vi "acquisitionSplitVolumes.vi"(4 "i-th volume":i32 min=0, 5 "volumeFirstFrame (from DAQ)":u32[](array[numeric]), 6 "frameCount (from Hamamatsu)":i32[](array[numeric]), 7 "frames":u16[][][](array[numeric])) -> (0 "numberOfFrames":i32, 1 "indexFirstFrame":i32, 2 "croppedFrameCount":u32[](array[numeric]), 3 "croppedFrames (volume)":u16[][][](array[numeric]))   [LabVIEW 2017]
doc: "Crop a single volume out of a continuous recording of frames, based on the two frame counts\nand the differentiator of the piezo monitor."
uses:
  globalUtilities.vi
panel:
  # "Crop a single volume out of a continuous recording of frames, based on the two frame counts\nand the differentiator of the piezo monitor."
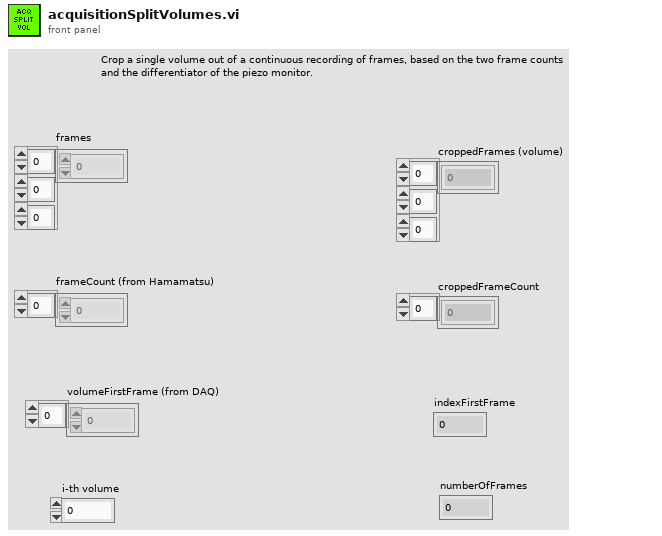
[diagram p1: front panel]
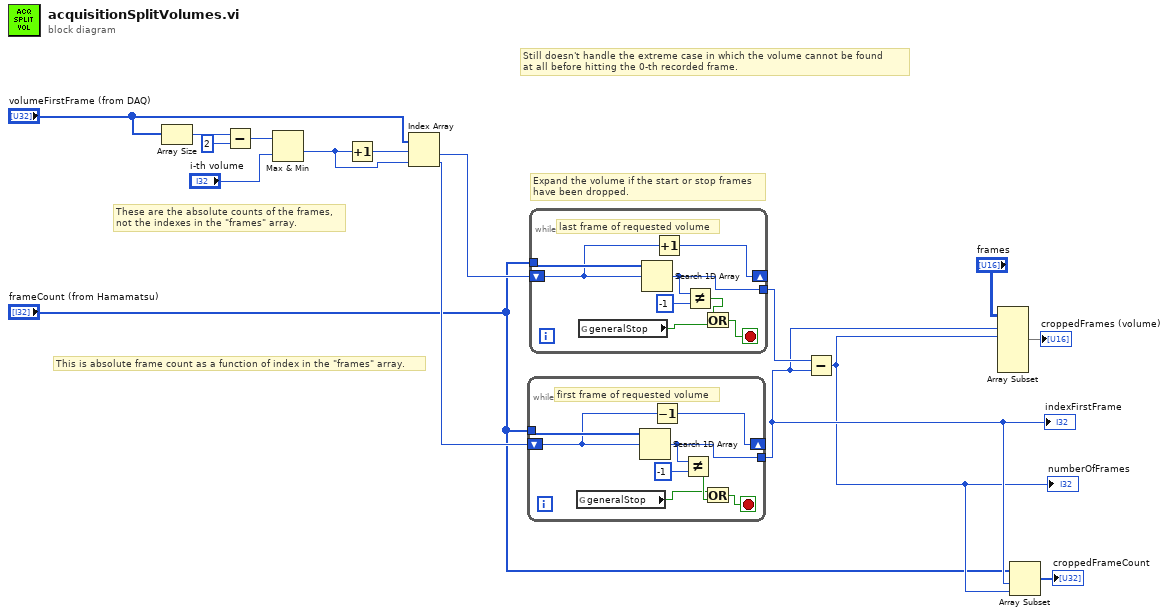
[diagram p0: block diagram]
diagram:
  # "Still doesn't handle the extreme case in which the volume cannot be found\nat all before hitting the 0-th recorded frame."
  # "Expand the volume if the start or stop frames\nhave been dropped."
  # "This is absolute frame count as a function of index in the \"frames\" array."
  # "These are the absolute counts of the frames,\nnot the indexes in the \"frames\" array."
  n1 = Array Size(array="volumeFirstFrame (from DAQ)") -> (size(s)=w14:i32)
  n2 = Subtract(x=w14, y=2) -> (x-y=w12:i32)
  n3 = Max & Min(x=w12, y="i-th volume") -> (min(x,y)=w10:i32)  [unwired: 1 out]
  n4 = Increment(x=w10) -> (x+1=w11:i32)
  n5 = Index Array(array="volumeFirstFrame (from DAQ)", index #1=w11, index #2=w10) -> (element #1=w6:u32, element #2=w7:u32)
  n6 = while {
    tunnel: "frameCount (from Hamamatsu)" -> [w24]
    shift-right: [w20] -> _
    shift-left: w7 -> [w22]
    tunnel: [w21] -> w4
    stop <- w17 stop-if-true
    # "first frame of requested volume"
    n7 = global read "globalUtilities.vi" "generalStop"() -> (w18:bool)
    n8 = Search 1D Array(1D array=w24, element=w22) -> (index of element=w21:i32)  [unwired: 1 in]
    n9 = Decrement(x=w22) -> (x-1=w20:u32)
    n10 = Not Equal?(x=w21, y=-1) -> (x != y?=w19:bool)
    n11 = Or(x=w18, y=w19) -> (x .or. y?=w17:bool)
  }
  "indexFirstFrame" <- w4
  n12 = while {
    tunnel: "frameCount (from Hamamatsu)" -> [w32]
    shift-right: [w28] -> _
    shift-left: w6 -> [w30]
    tunnel: [w29] -> w5
    stop <- w26 stop-if-true
    # "last frame of requested volume"
    n13 = global read "globalUtilities.vi" "generalStop"() -> (w25:bool)
    n14 = Search 1D Array(1D array=w32, element=w30) -> (index of element=w29:i32)  [unwired: 1 in]
    n15 = Increment(x=w30) -> (x+1=w28:u32)
    n16 = Not Equal?(x=w29, y=-1) -> (x != y?=w27:bool)
    n17 = Or(x=w27, y=w25) -> (x .or. y?=w26:bool)
  }
  n18 = Subtract(x=w5, y=w4) -> (x-y=w3:i32)
  "numberOfFrames" <- w3
  n19 = Array Subset(array="frames", index (dim 0)=w4, length (dim 0)=w3) -> (→"croppedFrames (volume)":u16[][][])  [unwired: 4 in]
  n20 = Array Subset(array="frameCount (from Hamamatsu)", index=w4, length=w3) -> (→"croppedFrameCount":i32[])
